vi "Test ManejoArchivos API.vi"() -> ()   [LabVIEW 2019]
doc: "ManejoArchivos API Tester."
uses:
  File Formats--enum.ctl
  <vilib>/Utility/error.llb/DialogType.ctl
  ManejoArchivos.lvlib
panel:
  out "Number Of Columns":i32
  in  "Get Number of Columns":bool
  in  "Close File":bool
  in  "Format":T1
  in  "Set File Format":bool
  in  "Data":dbl[](array[numeric])
  in  "Log Data":bool
  in  "Save Time Stamp":bool=TRUE
  in  "Delimiter":enum16{"Tab", "Coma"}(ring)
  in  "Set File Settings":bool
  in  "Path":path
  in  "Set File Path":bool
  in  "View File":bool
  in  "Headers":string[](array[string])
  in  "Set Column Headers":bool
  out "last error":errorcluster
  in  "Show Diagram on Init":bool
  in  "Show Block Diagram":bool
  in  "Stop Module":bool
  in  "Start Module":bool
  in  "Hide Module Panel":bool
  in  "Show Module Panel":bool
  out "Status":string
  out "Module Running?":bool
  # "This VI tests the API for the Module."
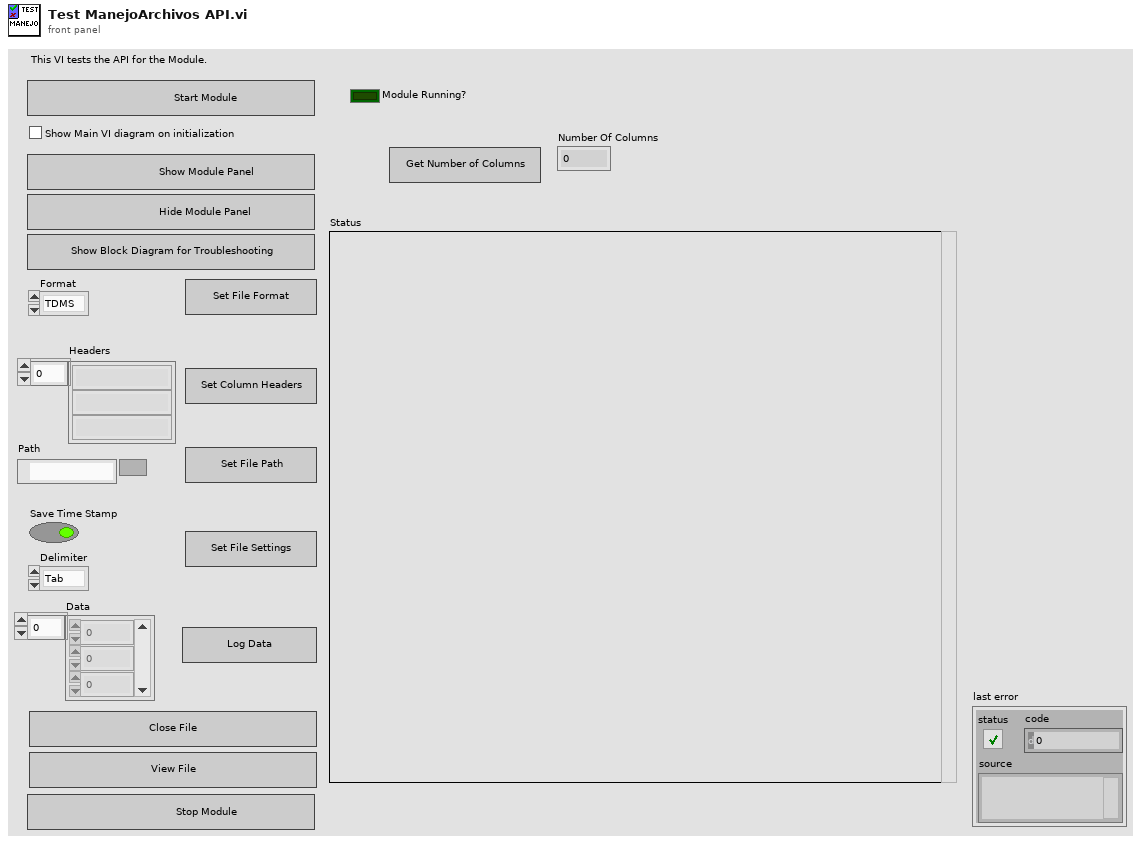
[diagram p1: front panel]
types:
  T1 = typedef "ManejoArchivos.lvlib/File Formats--enum.ctl" = enum16{"TDMS", "CSV"}
  T2 = typedef "ManejoArchivos.lvlib/Broadcast Events--cluster.ctl" = cluster{"Module Did Init":refnum<user-event>, "Status Updated":refnum<user-event>, "Error Reported":refnum<user-event>, "Module Did Stop":refnum<user-event>, "Update Module Execution Status":refnum<user-event>}
  T3 = typedef "DialogType.ctl" = u16
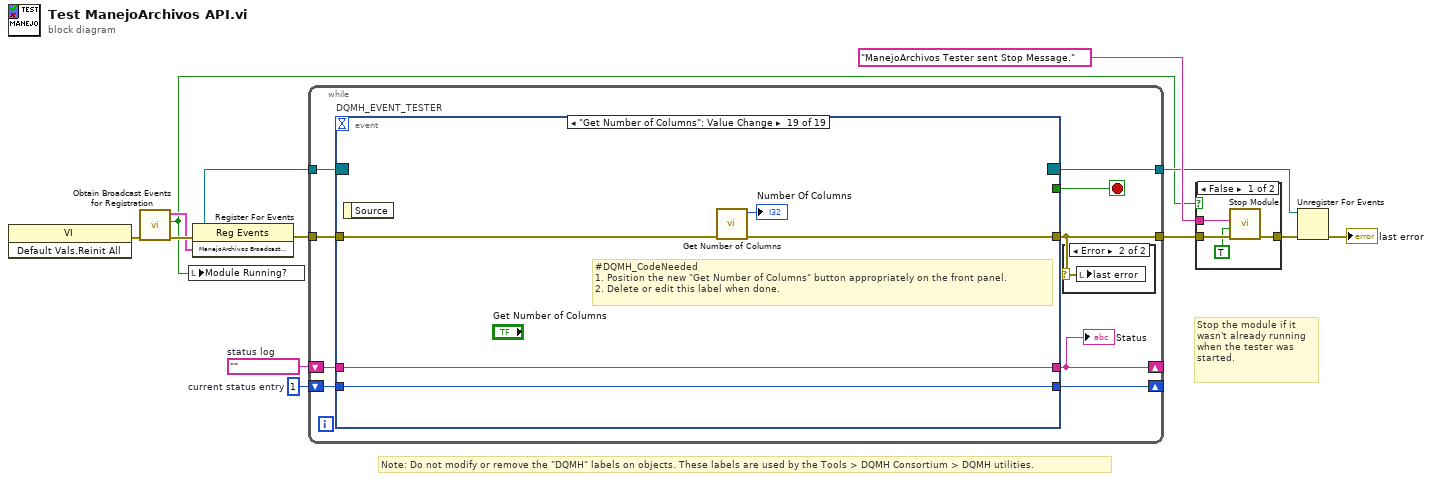
[diagram p0: block diagram]
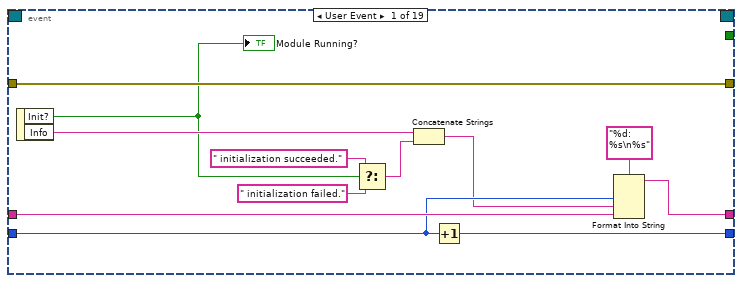
[diagram p4: hidden frame]
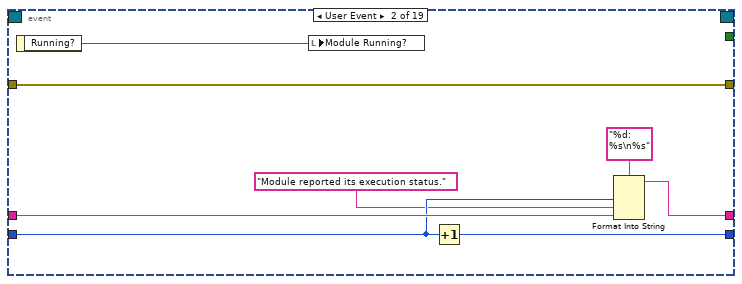
[diagram p5: hidden frame]
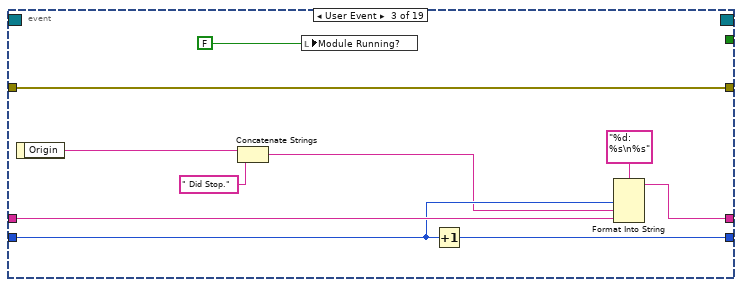
[diagram p6: hidden frame]
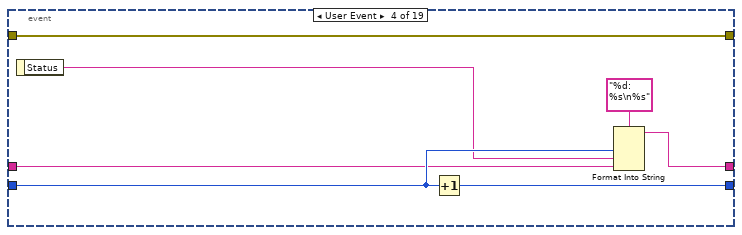
[diagram p7: hidden frame]
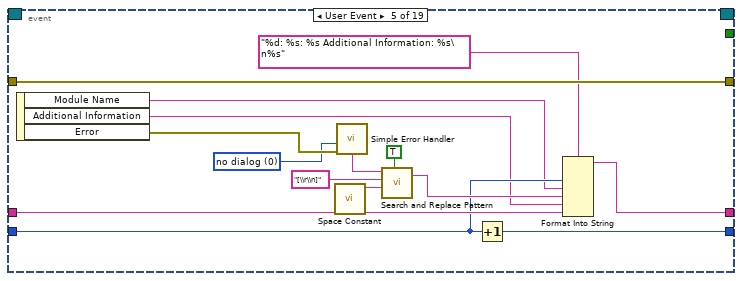
[diagram p8: hidden frame]
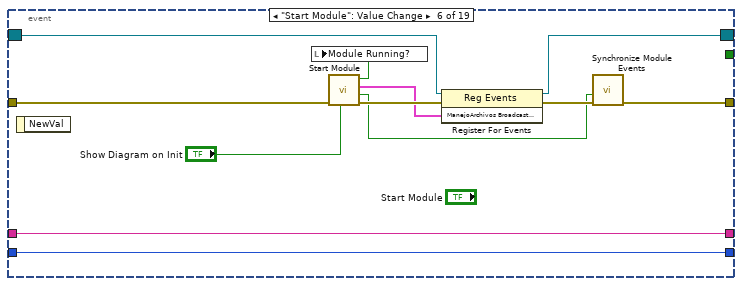
[diagram p9: hidden frame]
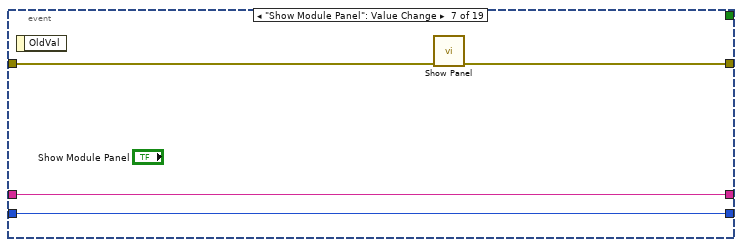
[diagram p10: hidden frame]
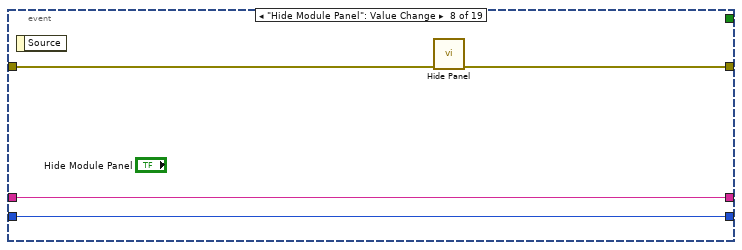
[diagram p11: hidden frame]
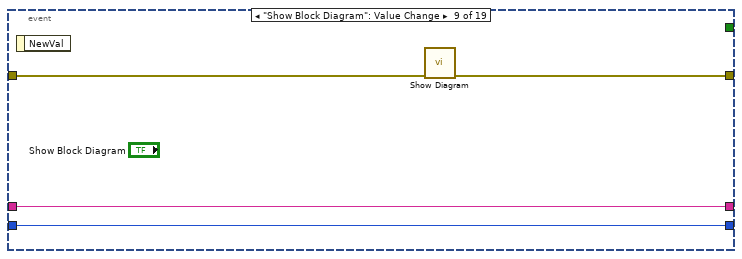
[diagram p12: hidden frame]
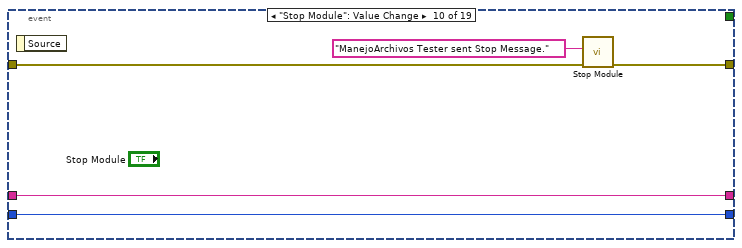
[diagram p13: hidden frame]
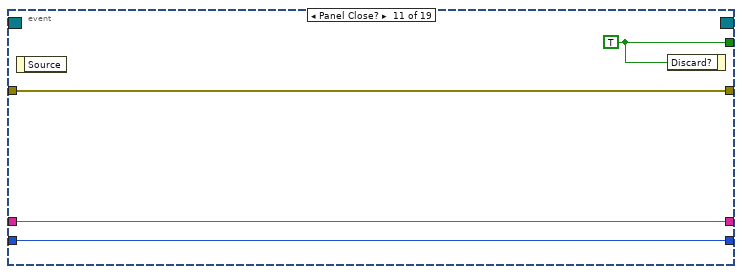
[diagram p14: hidden frame]
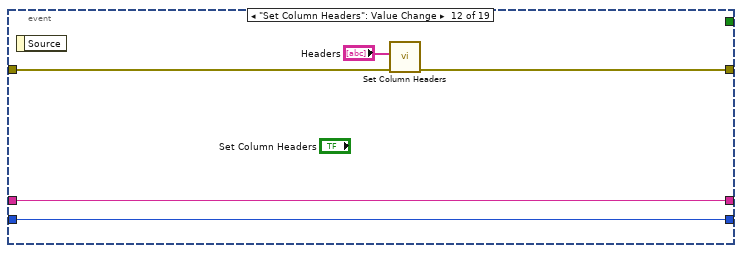
[diagram p15: hidden frame]
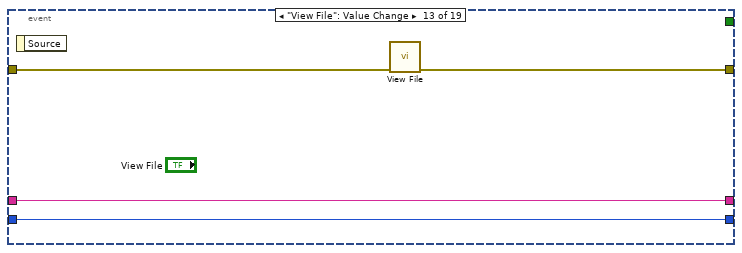
[diagram p16: hidden frame]
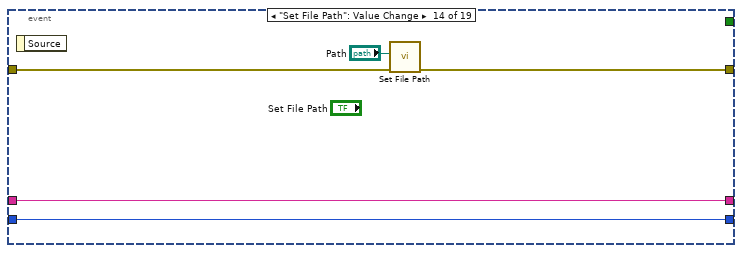
[diagram p17: hidden frame]
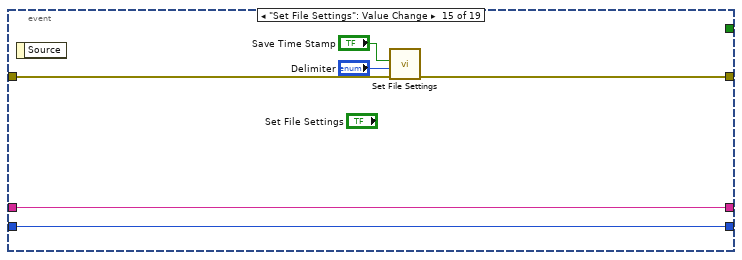
[diagram p18: hidden frame]
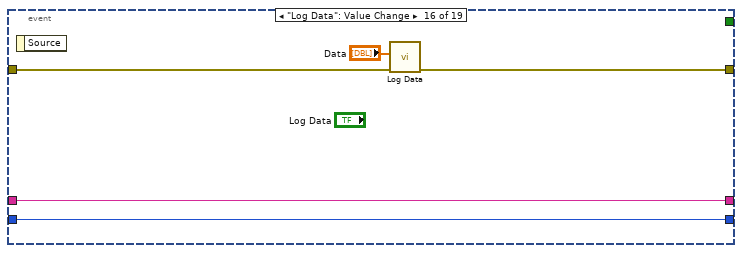
[diagram p19: hidden frame]
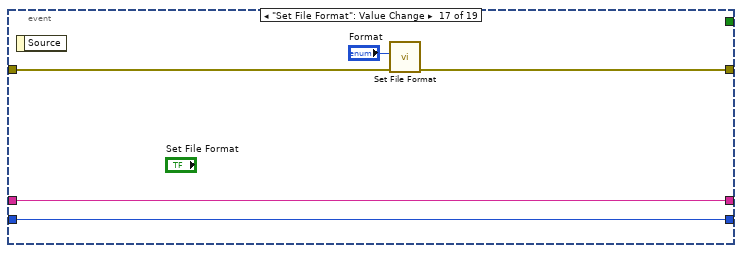
[diagram p20: hidden frame]
diagram:
  w5 = 1  # current status entry
  w6 = ""  # status log
  # "Stop the module if it wasn't already running when the tester was started."
  # "Note: Do not modify or remove the \"DQMH\" labels on objects. These labels are used by the Tools > DQMH Consortium > DQMH utilities."
  n1 = invoke class="VI" method="Default Vals.Reinit All"() -> (error out=w11:errorcluster)  [unwired: 3 in, 2 out]
  n2 = call "Obtain Broadcast Events for Registration.vi"("error in"=w11) -> ("error out"=w10:errorcluster, "Already running?"=w1:bool, "ManejoArchivos Broadcast Events"=w4:T2)  [unwired: 8 in]
  n3 = local write "Module Running?"(w1) -> ()
  n4 = register-events(error in=w10, w4) -> (reference out=w3:refnum<event-registration>, error out=w12:errorcluster)  [unwired: 1 in]
  n5 = while {
    tunnel: w3 -> [w20]
    tunnel: [w21] -> w9
    shift-right: [w16] -> _
    shift-left: w6 -> [w18]
    shift-right: [w17] -> _
    shift-left: w5 -> [w19]
    tunnel: w12 -> [w22]
    tunnel: [w15] -> w2
    stop <- w14 stop-if-true
    n6 = event "DQMH_EVENT_TESTER" shown="[18] \"Get Number of Columns\": Value Change" {
      selector: w20 -> [_ _ _ _ _ w79 _ _ _ _ _ _ _ _ _ _ _ _ _]
      dyn-events: [_ _ _ _ _ w78 _ _ _ _ _ _ _ _ _ _ _ _ _] -> w15
      timeout: _ -> [_ _ _ _ _ _ _ _ _ _ _ _ _ _ _ _ _ _ _]
      tunnel: [_ _ _ _ _ _ _ _ _ _ w107 _ _ _ _ _ _ _ _] -> w14
      tunnel: [w35 w43 w53 w60 w75 w85 w91 w95 w98 w104 w108 w112 w116 w121 w127 w132 w135 w139 w144] -> w21
      tunnel: w19 -> [w32 w40 w50 w56 w65 w82 w88 w92 w96 w101 w105 w110 w114 w119 w125 w130 w136 w140 w145]
      tunnel: w18 -> [w33 w41 w51 w55 w66 w83 w89 w93 w97 w102 w106 w111 w115 w120 w126 w131 w137 w141 w146]
      tunnel: [w30 w38 w48 w57 w64 w83 w89 w93 w97 w102 w106 w111 w115 w120 w126 w131 w137 w141 w146] -> w16
      tunnel: [w31 w39 w49 w59 w63 w82 w88 w92 w96 w101 w105 w110 w114 w119 w125 w130 w136 w140 w145] -> w17
      tunnel: w22 -> [w35 w43 w53 w60 w75 w84 w90 w94 w99 w103 w108 w113 w117 w122 w128 w133 w138 w142 w147]
      event User Event {
        n7 = event-data() -> ("Init?"=w27:bool, "Info"=w29:string)  [unwired: 1 in]
        "Module Running?" <- w27
        n8 = Select(t=" initialization succeeded.", s=w27, f=" initialization failed.") -> (s? t:f=w24:string)
        n9 = Concatenate Strings(w29, w24) -> (w28:string)
        n10 = Increment(x=w32) -> (x+1=w31:i32)
        n11 = Format Into String(format string="%d: %s\n%s", w32, w28, w33) -> (resulting string=w30:string)  [unwired: 2 in, 1 out]
      }
      event User Event {
        n12 = event-data() -> ("Running?"=w36:bool)  [unwired: 1 in]
        n13 = local write "Module Running?"(w36) -> ()
        n14 = Increment(x=w40) -> (x+1=w39:i32)
        n15 = Format Into String(format string="%d: %s\n%s", w40, "Module reported its execution status.", w41) -> (resulting string=w38:string)  [unwired: 2 in, 1 out]
      }
      event User Event {
        n16 = event-data() -> ("Origin"=w47:string)  [unwired: 1 in]
        n17 = Concatenate Strings(w47, " Did Stop.") -> (w46:string)
        n18 = local write "Module Running?"(FALSE ("Module Did Init?")) -> ()
        n19 = Increment(x=w50) -> (x+1=w49:i32)
        n20 = Format Into String(format string="%d: %s\n%s", w50, w46, w51) -> (resulting string=w48:string)  [unwired: 2 in, 1 out]
      }
      event User Event {
        n21 = event-data() -> ("Status"=w54:string)  [unwired: 1 in]
        n22 = Increment(x=w56) -> (x+1=w59:i32)
        n23 = Format Into String(format string="%d: %s\n%s", w56, w54, w55) -> (resulting string=w57:string)  [unwired: 2 in, 1 out]
      }
      event User Event {
        w67 = T3 0 items=["no dialog", "OK message", "continue or stop message", "OK message + warnings", "continue/stop + warnings"] ("type of dialog (OK msg:1)")
        n24 = event-data() -> ("Module Name"=w62:string, "Additional Information"=w61:string, "Error"=w74:errorcluster)  [unwired: 1 in]
        n25 = call <vilib>:"Space Constant.vi"() -> ("String"=w71:string)
        n26 = call <vilib>:"Simple Error Handler.vi"("type of dialog (OK msg:1)"=w67, "error in (no error)"=w74) -> ("message"=w68:string)  [unwired: 3 in, 4 out]
        n27 = call <vilib>:"Search and Replace Pattern.vi"("string"=w68, "regular expression (\"\")"="[\\r\\n]" ("regular expression (\"\")"), "replace string (\"\")"=w71, "replace all? (F)"=TRUE ("replace all CR/LF with spaces")) -> ("result string"=w69:string)  [unwired: 1 in, 1 out]
        n28 = Increment(x=w65) -> (x+1=w63:i32)
        n29 = Format Into String(format string="%d: %s: %s Additional Information: %s\n%s", w65, w62, w69, w61, w66) -> (resulting string=w64:string)  [unwired: 2 in, 1 out]
      }
      event "Start Module": Value Change {
        n30 = event-data() -> ()  [unwired: 1 in, 1 out]
        n31 = call "Start Module.vi"("Show Main VI Diagram on Init (F)"="Show Diagram on Init", "error in"=w84) -> ("error out"=w86:errorcluster, "Wait for Event Sync?"=w81:bool, "ManejoArchivos Broadcast Events"=w80:T2, "Module Was Already Running?"=w77:bool)  [unwired: 5 in, 1 out]
        n32 = local write "Module Running?"(w77) -> ()
        n33 = register-events(reference=w79, error in=w86, w80) -> (reference out=w78:refnum<event-registration>, error out=w87:errorcluster)
        n34 = call "Synchronize Module Events.vi"("error in"=w87, "Wait for Event Sync?"=w81) -> ("error out"=w85:errorcluster)  [unwired: 9 in]
      }
      event "Show Module Panel": Value Change {
        n35 = event-data() -> ()  [unwired: 1 in, 1 out]
        n36 = call "Show Panel.vi"("error in"=w90) -> ("error out"=w91:errorcluster)  [unwired: 10 in]
      }
      event "Hide Module Panel": Value Change {
        n37 = event-data() -> ()  [unwired: 1 in, 1 out]
        n38 = call "Hide Panel.vi"("error in"=w94) -> ("error out"=w95:errorcluster)  [unwired: 10 in]
      }
      event "Show Block Diagram": Value Change {
        n39 = event-data() -> ()  [unwired: 1 in, 1 out]
        n40 = call "Show Diagram.vi"("error in"=w99) -> ("error out"=w98:errorcluster)  [unwired: 10 in]
      }
      event "Stop Module": Value Change {
        n41 = event-data() -> ()  [unwired: 1 in, 1 out]
        n42 = call "Stop Module.vi"("error in"=w103, "Origin"="ManejoArchivos Tester sent Stop Message.") -> ("error out"=w104:errorcluster)  [unwired: 9 in]
      }
      event Panel Close? {
        w107 = TRUE ("Discard?")
        n43 = event-data() -> ()  [unwired: 1 in, 1 out]
        n44 = event-data("Discard?"=w107) -> ()  [unwired: 1 in, 1 out]
      }
      event "Set Column Headers": Value Change {
        n45 = event-data() -> ()  [unwired: 1 in, 1 out]
        n46 = call "Set Column Headers.vi"("error in"=w113, "Headers"="Headers") -> ("error out"=w112:errorcluster)  [unwired: 9 in]
      }
      event "View File": Value Change {
        n47 = event-data() -> ()  [unwired: 1 in, 1 out]
        n48 = call "View File.vi"("error in"=w117) -> ("error out"=w116:errorcluster)  [unwired: 10 in]
      }
      event "Set File Path": Value Change {
        n49 = event-data() -> ()  [unwired: 1 in, 1 out]
        n50 = call "Set File Path.vi"("error in"=w122, "Path"="Path") -> ("error out"=w121:errorcluster)  [unwired: 9 in]
      }
      event "Set File Settings": Value Change {
        n51 = event-data() -> ()  [unwired: 1 in, 1 out]
        n52 = call "Set File Settings.vi"("error in"=w128, "Delimiter"="Delimiter", "Save Time Stamp"="Save Time Stamp") -> ("error out"=w127:errorcluster)  [unwired: 8 in]
      }
      event "Log Data": Value Change {
        n53 = event-data() -> ()  [unwired: 1 in, 1 out]
        n54 = call "Log Data.vi"("error in"=w133, "Data"="Data") -> ("error out"=w132:errorcluster)  [unwired: 8 in, 1 out]
      }
      event "Set File Format": Value Change {
        n55 = event-data() -> ()  [unwired: 1 in, 1 out]
        n56 = call "Set File Format.vi"("error in"=w138, "Format"="Format") -> ("error out"=w135:errorcluster)  [unwired: 9 in]
      }
      event "Close File": Value Change {
        n57 = event-data() -> ()  [unwired: 1 in, 1 out]
        n58 = call "Close File.vi"("error in"=w142) -> ("error out"=w139:errorcluster)  [unwired: 10 in]
      }
      event "Get Number of Columns": Value Change {
        # "#DQMH_CodeNeeded\n1. Position the new \"Get Number of Columns\" button appropriately on the front panel.\n2. Delete or edit this label when done."
        n59 = event-data() -> ()  [unwired: 1 in, 1 out]
        n60 = call "Get Number of Columns.vi"("error in"=w147) -> ("error out"=w144:errorcluster, "Number Of Columns"=→"Number Of Columns":i32)  [unwired: 8 in, 1 out]
      }
    }
    "Status" <- w16
    n61 = case shown="Error" w21 {
      selector: w21 -> [_ w23]
      frame No Error {
      }
      frame Error {
        n62 = local write "last error"(w23) -> ()
      }
    }
  }
  n63 = case shown="False" w1 {
    tunnel: [w151 w152] -> w13
    tunnel: "ManejoArchivos Tester sent Stop Message." ("Origin") -> [w149 _]
    tunnel: w9 -> [w150 w152]
    frame False {
      n64 = call "Stop Module.vi"("error in"=w150, "Wait for Module to Stop? (F)"=TRUE ("Wait for Module to stop?"), "Origin"=w149) -> ("error out"=w151:errorcluster)  [unwired: 8 in]
    }
    frame True {
    }
  }
  n65 = Unregister For Events(event registration refnum=w2, error in=w13) -> (error out=→"last error":errorcluster)
